vi "LOC subConvertStringListToArrayOfStrings.vi"(1 "InputString":string) -> (0 "OutputArray":string[](array[string]))   [LabVIEW 2020, in "Localization_Tools.lvlib"]
uses:
  Localization_Tools.lvlib
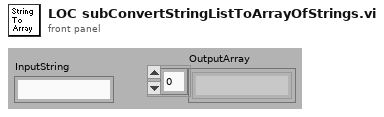
[diagram p1: front panel]
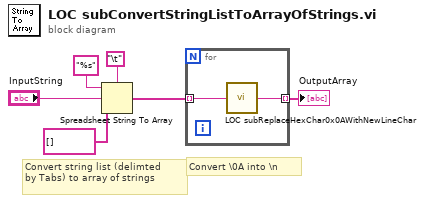
[diagram p0: block diagram]
diagram:
  # "Convert \\0A into \\n"
  # "Convert string list (delimted\nby Tabs) to array of strings"
  n1 = Spreadsheet String To Array(delimiter (Tab)="\t", format string="%s" ("delimiter (Tab)"), spreadsheet string="InputString", array type (2D Dbl)=string[] []) -> (array=w2:string[])
  n2 = for {
    tunnel: w2 -> [w8] mode=indexing
    tunnel: [w7] -> w1 mode=indexing
    n3 = call "LOC subReplaceHexChar0x0AWithNewLineChar.vi"("InputString"=w8) -> ("OutputString"=w7:string)
  }
  "OutputArray" <- w1
